vi "CommonSig-Apply Ramp.vi"   [LabVIEW 2020]
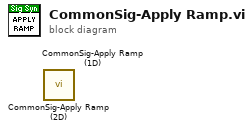
[diagram p0: block diagram]
diagram:
  n1 = call "CommonSig-Apply Ramp (2D).vi"() -> ()  [unwired: 14 in, 2 out]
  n2 = call "CommonSig-Apply Ramp (1D).vi"() -> ()  [unwired: 14 in, 2 out]
